vi "Reading the analog values and control the dc motor and a led.vi"() -> ()   [LabVIEW 2019]
uses:
  <vilib>/LabVIEW Interface for Arduino/Type Defs/Board Type.ctl
  <vilib>/LabVIEW Interface for Arduino/Type Defs/Connection Type.ctl
  <vilib>/LabVIEW Interface for Arduino/Type Defs/Pin Mode.ctl
  <vilib>/LabVIEW Interface for Arduino/LabVIEW Interface for Arduino.lvlib
panel:
  out "Slide":u8(slide) scale=0.0..255.0
  out "Tank":dbl(slide) scale=0.0..5.0
  in  "stop":bool
  in  "VISA resource":refnum<visa-resource-name>
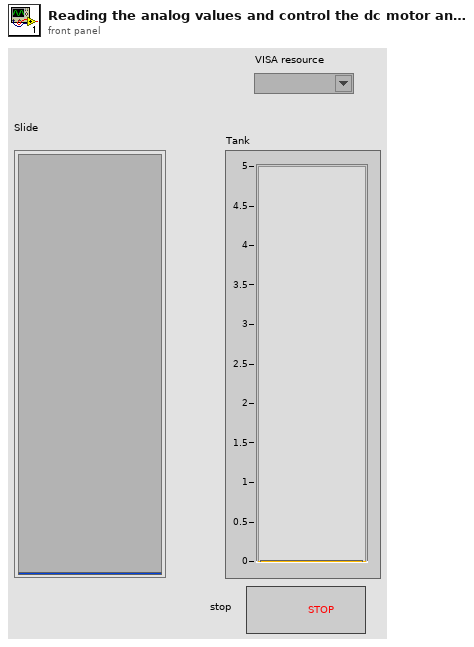
[diagram p1: front panel]
types:
  T1 = typedef "LabVIEW Interface for Arduino.lvlib/Pin Mode.ctl" = enum8{"Input", "Output"}
  T2 = typedef "LabVIEW Interface for Arduino.lvlib/Connection Type.ctl" = enum8{"USB / Serial", "XBEE", "BlueSmirf (Bluetooth)"}
  T3 = typedef "LabVIEW Interface for Arduino.lvlib/Board Type.ctl" = enum16{"Uno", "Dimuelanove w/Atmega 328", "Mega 2560"}
  T4 = typedef "LabVIEW Interface for Arduino.lvlib/Arduino Resource.ctl" = cluster{"VISA resource":refnum<visa-resource-name>, "Board Type":T3, "Connection Type":enum8{"USB / Serial"}, "Bytes Per Packet (15)":u8}
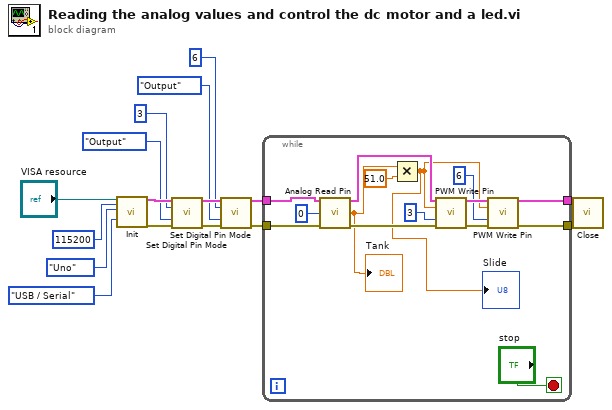
[diagram p0: block diagram]
diagram:
  n1 = call <vilib>:"Init.vi"("VISA resource"="VISA resource", "Baud Rate (115200)"=u32 115200, "Board Type (Uno)"=Board_Type."Uno", "Connection Type (USB/Serial)"=Connection_Type."USB / Serial") -> ("Arduino Resource"=w12:T4, "error out"=w10:errorcluster)  [unwired: 14 in]
  n2 = call <vilib>:"Set Digital Pin Mode.vi"("Arduino Resource"=w12, "Digital I/O Pin"=u8 3, "Pin Mode (Input)"=Pin_Mode."Output", "error in"=w10) -> ("Arduino Resource"=w11:T4, "error out"=w9:errorcluster)  [unwired: 10 in]
  n3 = call <vilib>:"Set Digital Pin Mode.vi"("Arduino Resource"=w11, "Digital I/O Pin"=u8 6, "Pin Mode (Input)"=Pin_Mode."Output", "error in"=w9) -> ("Arduino Resource"=w2:T4, "error out"=w1:errorcluster)  [unwired: 10 in]
  n4 = while {
    tunnel: [w26] -> w4
    tunnel: [w25] -> w3
    tunnel: w2 -> [w24]
    tunnel: w1 -> [w23]
    stop <- "stop" stop-if-true
    n5 = call <vilib>:"Analog Read Pin.vi"("Arduino Resource"=w24, "Analog Input Pin (0)"=u8 0, "error in"=w23) -> ("Arduino Resource"=w30:T4, "Voltage"=w18:dbl, "error out"=w29:errorcluster)  [unwired: 10 in]
    "Tank" <- w18
    n6 = Multiply(x=w18, y=51.0) -> (x*y=w17:dbl)
    "Slide" <- w17
    n7 = call <vilib>:"PWM Write Pin.vi"("Arduino Resource"=w30, "Duty Cycle (0 - 255)"=w17, "PWM Pin (3)"=u8 3, "error in"=w29) -> ("Arduino Resource"=w28:T4, "error out"=w27:errorcluster)  [unwired: 10 in]
    n8 = call <vilib>:"PWM Write Pin.vi"("Arduino Resource"=w28, "Duty Cycle (0 - 255)"=w17, "PWM Pin (3)"=u8 6, "error in"=w27) -> ("Arduino Resource"=w26:T4, "error out"=w25:errorcluster)  [unwired: 10 in]
  }
  n9 = call <vilib>:"Close.vi"("Arduino Resource"=w4, "error in"=w3) -> ()  [unwired: 13 in, 1 out]
